vi "Camera.TestLauncher.vi"() -> ()   [LabVIEW 2013]
doc: "JKI State Machine Objects (SMO) 1.0.0.5\nJKI - JKI\nCopyright (c) 2016, JKI"
uses:
  <vilib>/JKI/JKI SMO/SMO/Typedefs/SMOState --Enum.ctl
  Camera/Camera.lvclass
  <vilib>/JKI/JKI SMO/SMO/SMO.lvclass/SMO.ctl
  <vilib>/Utility/error.llb/DialogType.ctl
  <vilib>/JKI/JKI SMO/SMO/Private/ReftoDVR--SMO.vi
  <vilib>/JKI/JKI SMO/SMO/SMO.lvclass
  Microscope/Microscope.lvclass
panel:
  in  "Camera Type":string(combo)="Simulated"
  in  "Filepath":path
  in  "Save":bool
  out "Buffer":i32
  out "Image":picture
  out "State":T1
  in  "Grab":bool
  out "error out":errorcluster
  in  "Stop":bool
  # "Camera Test Launcher"
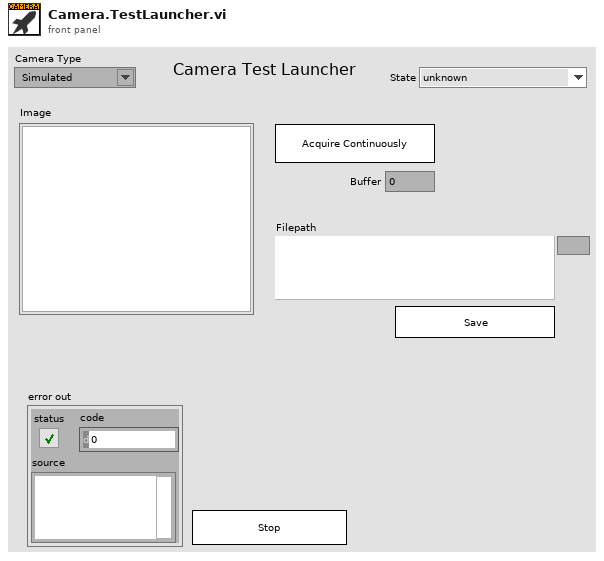
[diagram p1: front panel]
types:
  T1 = typedef "SMO.lvclass/SMOState --Enum.ctl" = enum16{"unknown", "Created", "Started", "Stopped"}
  T2 = typedef "Camera.lvclass/PublicEvents--Cluster.ctl" = cluster{"NewImage":refnum<user-event>, "ImageSaved":refnum<user-event>}
  T3 = typedef "SMO.lvclass/Public Events.ctl" = cluster{"Error":refnum<user-event>, "State":refnum<user-event>, "Reserve State":refnum<user-event>}
  T4 = cluster{"Event Registration Refnum":refnum<event-registration>}
  T5 = typedef "DialogType.ctl" = u16
  T6 = typedef "imagedata.ctl" = cluster{"image type":i32, "image depth":i32, "image":u8[], "mask":u8[], "colors":u32[], "Rectangle":cluster{"left":i16, "top":i16, "right":i16, "bottom":i16}}
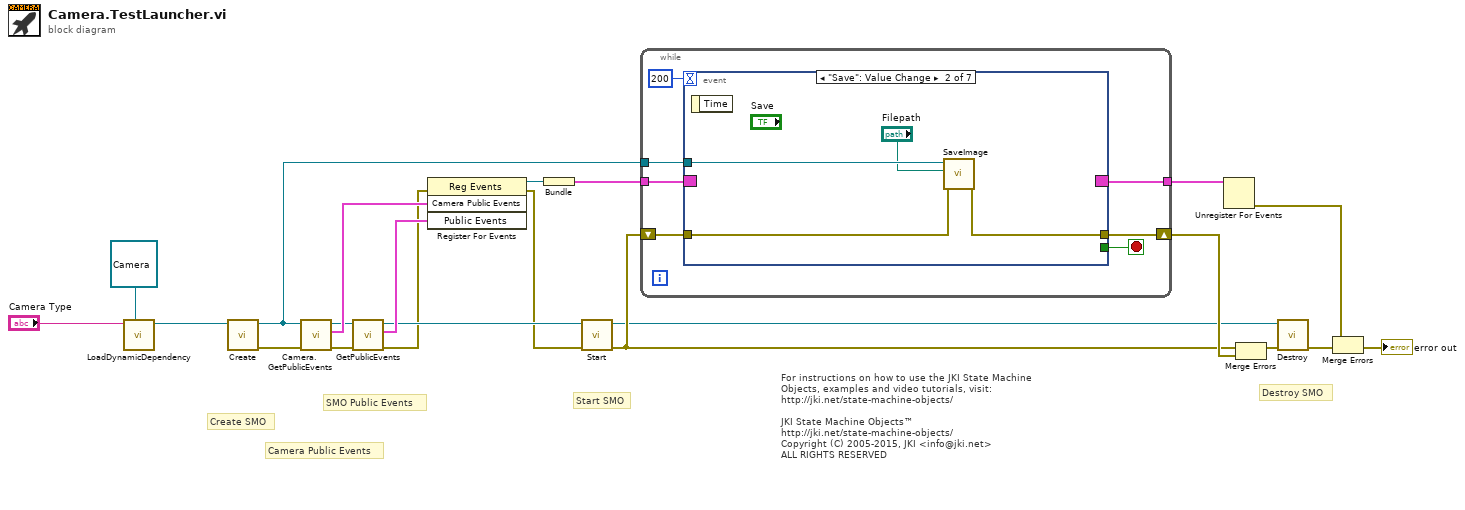
[diagram p0: block diagram]
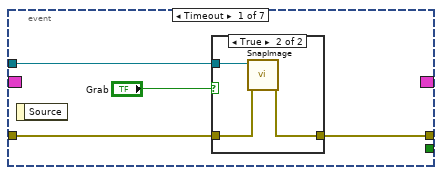
[diagram p2: hidden frame]
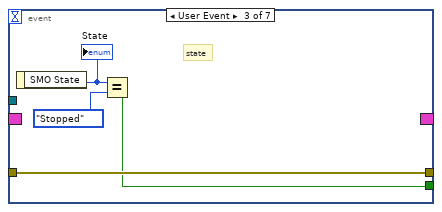
[diagram p4: hidden frame]
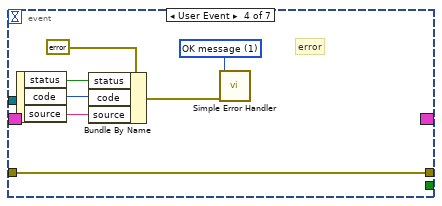
[diagram p5: hidden frame]
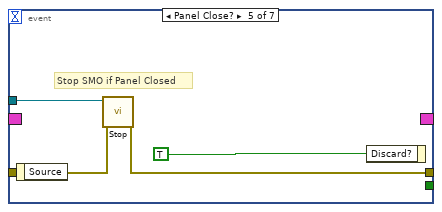
[diagram p6: hidden frame]
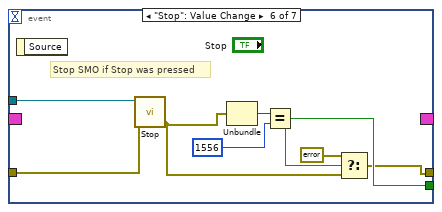
[diagram p7: hidden frame]
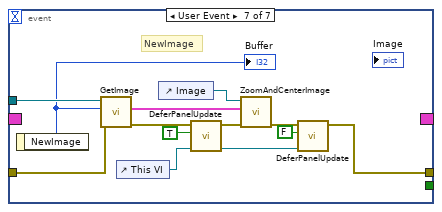
[diagram p8: hidden frame]
diagram:
  # "SMO Public Events"
  # "For instructions on how to use the JKI State Machine Objects, examples and video tutorials, visit:\nhttp://jki.net/state-machine-objects/\n\nJKI State Machine Objects™\nhttp://jki.net/state-machine-objects/\nCopyright (C) 2005-2015, JKI <info@jki.net>\nALL RIGHTS RESERVED"
  # "Camera Public Events"
  # "Start SMO"
  # "Destroy SMO"
  # "Create SMO"
  n1 = call "LoadDynamicDependency.vi"("SMO in"=refnum<class "Camera.lvclass"> refnum ("SMO.Template.lvclass"), "Camera"="Camera Type") -> ("SMO out"=w1:refnum<class "Camera.lvclass">)  [unwired: 8 in, 1 out]
  n2 = call <vilib>:"Create.vi"("SMO"=w1) -> ("error out"=w5:errorcluster, "SMO out"=w4:refnum<class "Camera.lvclass">)  [unwired: 8 in, 1 out]
  n3 = call "Camera.GetPublicEvents.vi"("error in (no error)"=w5, "Camera"=w4) -> ("error out"=w12:errorcluster, "Camera Public Events"=w15:T2, "Camera out"=w13:refnum<class "Camera.lvclass">)  [unwired: 7 in]
  n4 = call <vilib>:"GetPublicEvents.vi"("error in (no error)"=w12, "SMO"=w13) -> ("error out"=w9:errorcluster, "Public Events"=w11:T3, "SMO out"=w10:refnum<class "Camera.lvclass">)  [unwired: 7 in]
  n5 = register-events(error in=w9, w15, w11) -> (reference out=w14:refnum<event-registration>, error out=w8:errorcluster)  [unwired: 1 in]
  n6 = Bundle("Event Registration Refnum"=w14) -> (w21:T4)  [unwired: 1 in]
  n7 = call <vilib>:"Start.vi"("error in (no error)"=w8, "SMO"=w10) -> ("error out"=w16:errorcluster, "SMO out"=w6:refnum<class "Camera.lvclass">)  [unwired: 8 in]
  n8 = while {
    shift-right: [w28] -> w20
    shift-left: w16 -> [w27]
    tunnel: w21 -> [w26]
    tunnel: [w25] -> w22
    tunnel: w4 -> [w24]
    stop <- w29 stop-if-true
    n9 = event shown="[1] \"Save\": Value Change" {
      selector: w26 -> [_ _ _ _ _ _ _]
      dyn-events: [_ _ _ _ _ _ _] -> w25
      timeout: 200 -> [_ _ _ _ _ _ _]
      tunnel: [_ _ w42 _ _ w60 _] -> w29
      tunnel: w24 -> [w33 w41 _ _ w56 w64 w77]
      tunnel: [w31 w39 w45 w52 w55 w57 w67] -> w28
      tunnel: w27 -> [w32 w40 w45 w52 w54 w63 w75]
      event Timeout {
        n10 = event-data() -> ()  [unwired: 1 in, 1 out]
        n11 = case shown="True" "Grab" {
          tunnel: w33 -> [_ w37]
          tunnel: w32 -> [w34 w36]
          tunnel: [w34 w35] -> w31
          frame False {
          }
          frame True {
            n12 = call "SnapImage.vi"("error in (no error)"=w36, "Camera"=w37) -> ("error out"=w35:errorcluster)  [unwired: 7 in, 2 out]
          }
        }
      }
      event "Save": Value Change {
        n13 = event-data() -> ()  [unwired: 1 in, 1 out]
        n14 = call "SaveImage.vi"("error in (no error)"=w40, "Path"="Filepath", "Camera"=w41) -> ("error out"=w39:errorcluster)  [unwired: 7 in, 1 out]
      }
      event User Event {
        # "state"
        n15 = event-data() -> ("SMO State"=w44:T1)  [unwired: 1 in]
        "State" <- w44
        n16 = Equal?(x=w44, y=SMOState_--Enum."Stopped") -> (x = y?=w42:bool)
      }
      event User Event {
        w46 = T5 1 items=["no dialog", "OK message", "continue or stop message", "OK message + warnings", "continue/stop + warnings"] ("type of dialog (OK msg:1)")
        # "error"
        n17 = event-data() -> ("status"=w50:bool, "code"=w49:i32, "source"=w48:string)  [unwired: 1 in]
        n18 = Bundle By Name(cluster=errorcluster {"status"=FALSE, "code"=0, "source"=""} ("error out"), "status"=w50, "code"=w49, "source"=w48) -> (w47:errorcluster)
        n19 = call <vilib>:"Simple Error Handler.vi"("type of dialog (OK msg:1)"=w46, "error in (no error)"=w47) -> ()  [unwired: 3 in, 5 out]
      }
      event Panel Close? {
        # "Stop SMO if Panel Closed"
        n20 = event-data() -> ()  [unwired: 1 in, 1 out]
        n21 = call <vilib>:"Stop.vi"("error in (no error)"=w54, "SMO"=w56) -> ("error out"=w55:errorcluster)  [unwired: 8 in, 1 out]
        n22 = event-data("Discard?"=TRUE ("OK")) -> ()  [unwired: 1 in, 1 out]
      }
      event "Stop": Value Change {
        # "Stop SMO if Stop was pressed"
        n23 = event-data() -> ()  [unwired: 1 in, 1 out]
        n24 = call <vilib>:"Stop.vi"("error in (no error)"=w63, "SMO"=w64) -> ("error out"=w59:errorcluster)  [unwired: 8 in, 1 out]
        n25 = Unbundle(w59) -> ("code"=w62:i32)  [unwired: 2 out]
        n26 = Equal?(x=w62, y=1556 ("specific error code to clear (0: all)")) -> (x = y?=w60:bool)
        n27 = Select(t=errorcluster {"status"=FALSE, "code"=0, "source"=""}, s=w60, f=w59) -> (s? t:f=w57:errorcluster)
      }
      event User Event {
        # "NewImage"
        n28 = event-data() -> ("NewImage"=w76:i32)  [unwired: 1 in]
        "Buffer" <- w76
        n29 = call "GetImage.vi"("error in (no error)"=w75, "Get Image (-1: latest)"=w76, "Camera"=w77) -> ("error out"=w70:errorcluster, "image data"=w69:T6)  [unwired: 6 in, 1 out]
        n30 = control-ref of="This VI"() -> (w66:refnum<vi>)
        n31 = control-ref of="Image"() -> (w68:refnum<vi>)
        n32 = call "DeferPanelUpdate.vi"("VI in"=w66, "defer panel updates"=TRUE, "error in (no error)"=w70) -> ("VI out"=w65:refnum<vi>, "error out"=w72:errorcluster)  [unwired: 7 in]
        n33 = call "ZoomAndCenterImage.vi"("error in (no error)"=w72, "image data"=w69, "Picture Ref"=w68) -> ("error out"=w71:errorcluster)  [unwired: 8 in]
        n34 = call "DeferPanelUpdate.vi"("VI in"=w65, "defer panel updates"=FALSE, "error in (no error)"=w71) -> ("error out"=w67:errorcluster)  [unwired: 7 in, 1 out]
      }
    }
  }
  n35 = Unregister For Events(event registration refnum=w22) -> (error out=w19:errorcluster)  [unwired: 1 in]
  n36 = Merge Errors(w16, w20) -> (w7:errorcluster)
  n37 = call <vilib>:"Destroy.vi"("error in (no error)"=w7, "SMO"=w6) -> ("error out"=w17:errorcluster)  [unwired: 9 in]
  n38 = Merge Errors(w19, w17) -> (→"error out":errorcluster)
